vi "find offset by percent.vi"(2 "low %":dbl format="%.2f", 3 "orders":u8[][](array[numeric])) -> (1 "offset":dbl format="%.2f")   [LabVIEW 2017]
uses:
  <vilib>/Analysis/NI_AALBase.lvlib
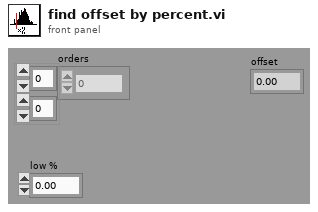
[diagram p1: front panel]
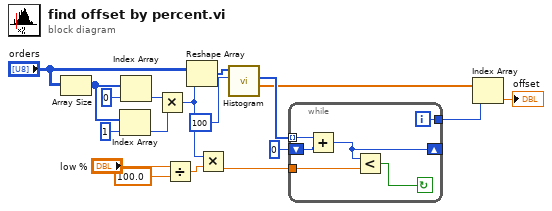
[diagram p0: block diagram]
diagram:
  n1 = Array Size(array="orders") -> (size(s)=w16:i32[])
  n2 = Index Array(array=w16, index=1 ("Index")) -> (element=w12:i32)
  n3 = Index Array(array=w16, index=0 ("Index")) -> (element=w13:i32)
  n4 = Multiply(x=w13, y=w12) -> (x*y=w10:i32)
  n5 = Divide(x="low %", y=100.0) -> (x/y=w2:dbl)
  n6 = Reshape Array("orders", w10) -> (w18:u8[])
  n7 = Multiply(x=w10, y=w2) -> (x*y=w7:dbl)
  n8 = call <vilib>:"Histogram.vi"("intervals"=100, "X"=w18) -> ("X Values"=w6:dbl[], "Histogram: h(x)"=w8:i32[])  [unwired: 6 in, 2 out]
  n9 = while {
    tunnel: [w19] -> w5
    tunnel: w7 -> [w21]
    tunnel: w8 -> [w23] mode=indexing
    shift-left: 0 -> [w24]
    shift-right: [w22] -> _
    i -> [w19]
    stop <- w20 continue-if-true
    n10 = Add(x=w23, y=w24) -> (x+y=w22:i32)
    n11 = Less?(x=w22, y=w21) -> (x < y?=w20:bool)
  }
  n12 = Index Array(array=w6, index=w5) -> (element=→"offset":dbl)
